vi "Main.vi"() -> ()   [LabVIEW 2021]
doc: "The myRIO Project template acquires acceleration data from the onboard accelerometer and displays the changes of acceleration values in a waveform chart."
uses:
  <vilib>/myRIO/Instrument Drivers/Onboard IO/I2C/typedefs/I2C User Configuration.ctl
  <vilib>/myRIO/Instrument Drivers/Onboard IO/I2C/typedefs/I2C Transfer Rate.ctl
  <vilib>/myRIO/Instrument Drivers/Onboard IO/I2C/typedefs/I2C Reference.ctl
  <vilib>/myRIO/Common/Instrument Driver Framework/Utilities/typedefs/myRIO Generic Hardware Reference.ctl
  <vilib>/myRIO/Common/Instrument Driver Framework/Utilities/typedefs/Hardware Version Enum.ctl
  <vilib>/myRIO/Common/Instrument Driver Framework/Utilities/typedefs/myRIO v1.0 Reference.ctl
  <vilib>/myRIO/Common/Instrument Driver Framework/Utilities/typedefs/Generic FPGA Reference.ctl
  <vilib>/myRIO/Common/Instrument Driver Framework/myRIO v1.0/I2C/typedefs/I2C Channels Enum.ctl
  <vilib>/myRIO/Instrument Drivers/Onboard IO/I2C/typedefs/I2C Configuration.ctl
  <vilib>/userDefined/High Color/nirio_resource_hc.ctl
  <vilib>/Platform/TimedLoop/XDataNode/timing_clust.ctl
  <vilib>/Platform/TimedLoop/XDataNode/nitl_modes.ctl
  <vilib>/Platform/TimedLoop/XDataNode/wakeup.ctl
  <vilib>/myRIO/Instrument Drivers/Onboard IO/PWM/typedefs/PWM Reference.ctl
  <vilib>/myRIO/Common/Instrument Driver Framework/myRIO v1.0/PWM/typedefs/PWM Channels Enum.ctl
  <vilib>/myRIO/Instrument Drivers/Onboard IO/PWM/typedefs/PWM Configuration.ctl
  <vilib>/myRIO/Common/Instrument Driver Framework/Utilities/vis/Is FPGA Ref Available.vi
  <vilib>/myRIO/Common/Instrument Driver Framework/myRIO v1.0/I2C/vis/myRIO v1.1 Open I2C.vi
  <vilib>/myRIO/Instrument Drivers/Onboard IO/I2C/vis/Configure.vi
  <vilib>/myRIO/Instrument Drivers/Onboard IO/I2C/vis/Write.vi
  <vilib>/myRIO/Instrument Drivers/Onboard IO/I2C/vis/Read.vi
  <vilib>/myRIO/Instrument Drivers/Onboard IO/I2C/vis/Write Read.vi
  <vilib>/myRIO/Common/Instrument Driver Framework/myRIO v1.0/PWM/vis/myRIO v1.1 Open PWM.vi
  <vilib>/myRIO/Instrument Drivers/Onboard IO/PWM/vis/Set Duty Cycle and Frequency.vi
  <vilib>/myRIO/Common/Instrument Driver Framework/Utilities/vis/Validate Channels.vi
  <vilib>/myRIO/Common/Instrument Driver Framework/myRIO v1.0/I2C/vis/myRIO v1.0 Reserve I2C.vi
  <vilib>/myRIO/Common/Instrument Driver Framework/myRIO v1.0/PWM/vis/myRIO v1.0 Reserve PWM.vi
  <vilib>/myRIO/Common/Instrument Driver Framework/myRIO v1.0/I2C/vis/myRIO v1.0 Build MUX Configuration I2C.vi
  <vilib>/myRIO/Common/Instrument Driver Framework/myRIO v1.0/Resource Manager/vis/myRIO v1.0 Reserve Channel List.vi
  <vilib>/myRIO/Common/Instrument Driver Framework/myRIO v1.0/PWM/vis/myRIO v1.0 Build MUX Configuration PWM.vi
  <vilib>/myRIO/Common/Instrument Driver Framework/myRIO v1.0/Resource Manager/vis/myRIO v1.0 Create Configuration List.vi
  <vilib>/myRIO/Common/Instrument Driver Framework/myRIO v1.0/Resource Manager/vis/myRIO v1.0 Reserve Channel.vi
  <vilib>/myRIO/Common/Instrument Driver Framework/myRIO v1.0/Resource Manager/vis/myRIO v1.0 Unreserve Channel.vi
  <vilib>/myRIO/Common/Instrument Driver Framework/myRIO v1.0/Resource Manager/vis/myRIO v1.0 Build Mutex Name.vi
  <vilib>/Utility/VariantDataType/GetNumericInfo.vi
  <vilib>/Utility/error.llb/Error Cluster From Error Code.vi
  <vilib>/myRIO/Common/Instrument Driver Framework/myRIO v1.0/myRIO v1.1 Open.vi
  <vilib>/myRIO/Common/Instrument Driver Framework/Utilities/vis/IO Manager.vi
  <vilib>/myRIO/Common/Instrument Driver Framework/Utilities/vis/Configuration Manager.vi
  <vilib>/myRIO/Common/Instrument Driver Framework/myRIO v1.0/Resource Manager/vis/myRIO v1.0 Configure IO.vi
  <vilib>/myRIO/Common/Instrument Driver Framework/myRIO v1.0/myRIO v1.0 Close.vi
  <vilib>/myRIO/Common/Instrument Driver Framework/myRIO v1.0/I2C/vis/myRIO v1.0 Configure I2C.vi
  <vilib>/myRIO/Common/Instrument Driver Framework/myRIO v1.0/I2C/vis/myRIO v1.0 Write I2C.vi
  <vilib>/myRIO/Common/Instrument Driver Framework/myRIO v1.0/I2C/vis/myRIO v1.0 Read I2C.vi
  <vilib>/myRIO/Common/Instrument Driver Framework/myRIO v1.0/PWM/vis/myRIO v1.0 Write PWM.vi
  <vilib>/Skyline/Tag/Wrapper/Wrapper_class/Close Tag (Multiple).vi
  <vilib>/Skyline/Tag/Wrapper/Wrapper_class/NI Skyline Tag.lvclass
  <vilib>/myRIO/Express VI/Onboard IO/I2C/I2C Express VI.xnode
  <vilib>/myRIO/Instrument Drivers/Onboard IO/I2C/vis/myRIO I2C Open.xnode
  <vilib>/platform/TimedLoop/XDataNode/XDataNode.xnode
  <vilib>/myRIO/Express VI/Onboard IO/PWM/PWM Express VI.xnode
  <vilib>/myRIO/Instrument Drivers/Onboard IO/PWM/vis/myRIO PWM Open.xnode
  <vilib>/myRIO/Instrument Drivers/Onboard IO/I2C/I2C.lvlib
  <vilib>/Platform/TimedLoop/XDataNode/XDNodeRunTimeDep.lvlib
  <vilib>/myRIO/Instrument Drivers/Onboard IO/PWM/PWM.lvlib
panel:
  out "Warmer\nON":bool
  out "Coffee Temp (°F)":dbl
  out "Error":errorcluster
  out "HOT\nSurface":bool
  out "Plate Temp (°F)":dbl
  out "Surface Danger Level":string
  out "Set-Temp-Slider":dbl(slide) scale=80.0..180.0
  out "Temp-Chart":T1(graph)
  in  "stop":bool
  # "Nice Warm Coffee"
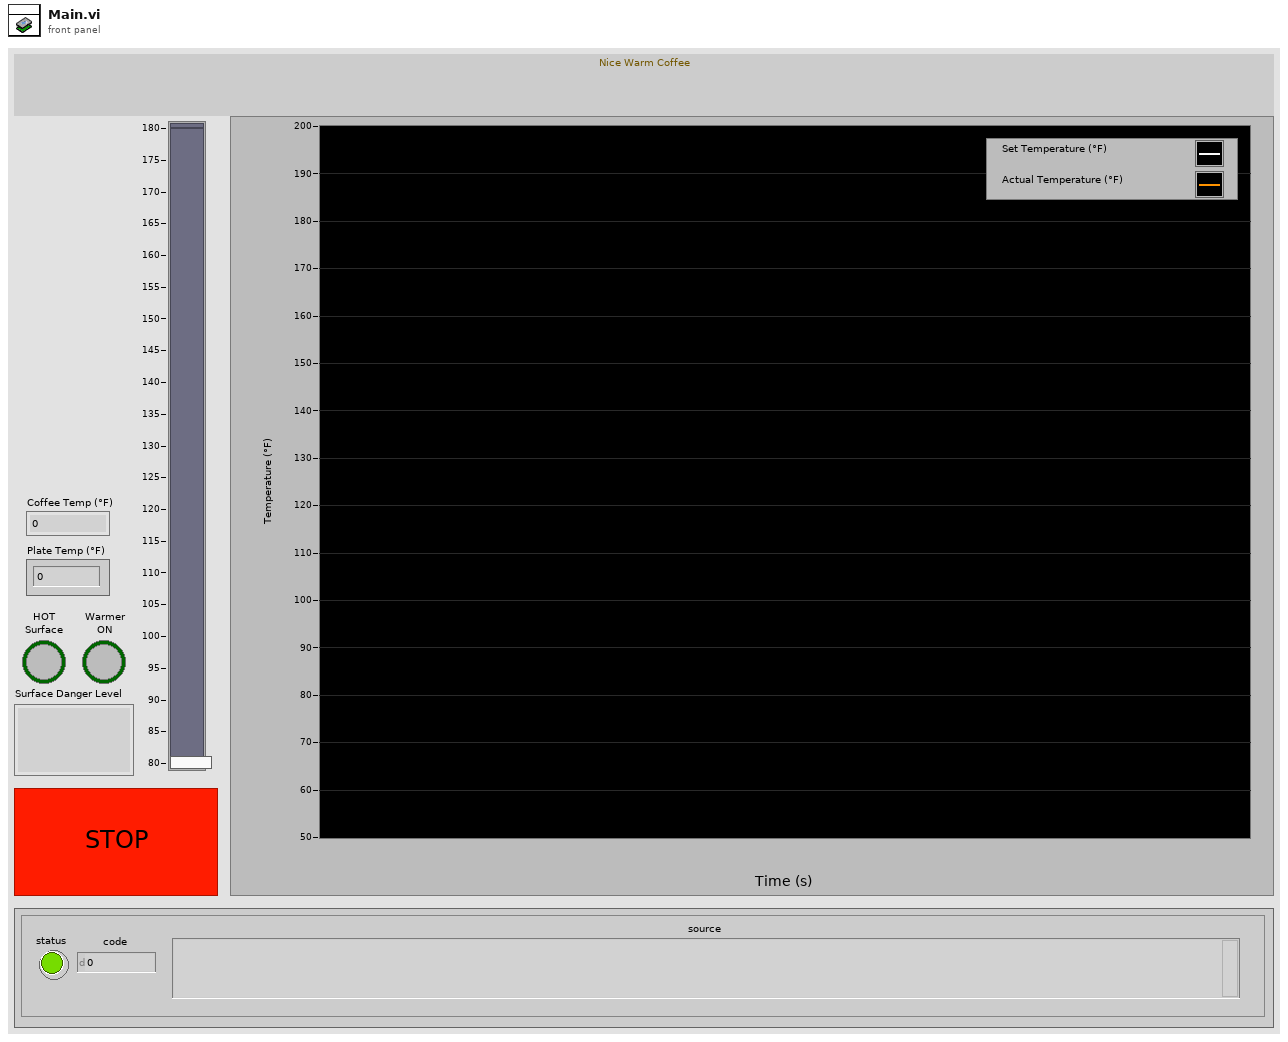
[diagram p1: front panel]
types:
  T1 = cluster{"[0]":dbl, "[1]":dbl, "[2]":dbl, "[3]":dbl, "[4]":dbl, "[5]":dbl, "[6]":dbl, "[7]":dbl, "[8]":dbl}
  T2 = typedef "XDNodeRunTimeDep.lvlib/timing_clust.ctl" = cluster{"Expected End [f-1]":u64, "Actual End [f-1]":u64, "Finished Late? [f-1]":bool, "Expected End [i-1]":u64, "Actual End [i-1]":u64, "Finished Late? [i-1]":bool, "Expected Start [i]":u64, "Actual Start [i]":u64, "Expected Start [f]":u64, "Actual Start [f]":u64, "Source Name":string, "Structure Name":string, "Period":i64, "Deadline":i64, "Offset":i64, "Start":i64, "Priority":i32, "Timeout":i32, "Mode":T3, "Wakeup Reason":T4, "Error":errorcluster, "Source Type":string, "Secondary Source Type":string, "Global End Time":u64, "Global Start Time":u64, "Frame Duration":u64, "Iteration Duration":u64, "Assigned CPU":i32, "I/O Scan Engine Mode":u32}
  T3 = typedef "XDNodeRunTimeDep.lvlib/nitl_modes.ctl" = enum32{"No Change", "Process missed periods, maintain original phase", "Discard missed periods, maintain original phase", "Process missed periods, ignore original phase", "Discard missed periods, ignore original phase"}
  T4 = typedef "XDNodeRunTimeDep.lvlib/wakeup.ctl" = enum32{"Normal", "Aborted", "Asynchronous wakeup", "Timing source error", "Timed loop error", "Timeout"}
  T5 = typedef "PWM.lvlib/PWM Reference.ctl" = cluster{"myRIO Reference":T6, "PWM Channels Enum":T10, "PWM Configuration":T11}
  T6 = typedef "myRIO Generic Hardware Reference.ctl" = cluster{"myRIO Model":T7, "myRIO Hardware Reference":T8}
  T7 = typedef "Hardware Version Enum.ctl" = enum16{"Unknown", "myRIO-1900", "myRIO-1950", "roboRIO", "NI ELVIS RIO CM", "ELVIS III"}
  T8 = typedef "myRIO v1.0 Reference.ctl" = cluster{"Generic FPGA Reference":T9, "Allow multiple opens":bool}
  T9 = typedef "Generic FPGA Reference.ctl" = refnum<k20>
  T10 = typedef "PWM Channels Enum.ctl" = enum16{"Not Connected", "C/PWM0", "C/PWM1", "A/PWM0", "A/PWM1", "A/PWM2", "A/PWM3", "A/PWM4", "A/PWM5", "A/PWM6", "A/PWM7", "A/PWM8", "A/PWM9", "A/PWM10", "A/PWM11", "A/PWM12", "A/PWM13", "A/PWM14", "A/PWM15", "A/PWM16", "A/PWM17", "A/PWM18", "A/PWM19", "B/PWM0", "B/PWM1", "B/PWM2", "B/PWM3", "B/PWM4", "B/PWM5", "B/PWM6", "B/PWM7", "B/PWM8", "B/PWM9", "B/PWM10", "B/PWM11", "B/PWM12", "B/PWM13", "B/PWM14", "B/PWM15", "B/PWM16", "B/PWM17", "B/PWM18", "B/PWM19", "PWM/PWM0", "PWM/PWM1", "PWM/PWM2", "PWM/PWM3", "PWM/PWM4", "PWM/PWM5", "PWM/PWM6", "PWM/PWM7", "PWM/PWM8", "PWM/PWM9"}
  T11 = typedef "PWM.lvlib/PWM Configuration.ctl" = cluster{"Frequency":dbl, "Duty Cycle":dbl}
  T12 = typedef "nirio_resource_hc.ctl" = tag
  T13 = typedef "I2C.lvlib/I2C Reference.ctl" = cluster{"myRIO Reference":T6, "I2C Channels Enum":T14, "I2C Configuration":T15}
  T14 = typedef "I2C Channels Enum.ctl" = enum16{"Not Connected", "A/I2C", "B/I2C", "I2C/I2C"}
  T15 = typedef "I2C.lvlib/I2C Configuration.ctl" = cluster{"I2C Transfer Rate":T16}
  T16 = typedef "I2C.lvlib/I2C Transfer Rate.ctl" = enum16{"Standard mode (100 kbps)", "Fast mode (400 kbps)"}
  T17 = typedef "I2C.lvlib/I2C User Configuration.ctl" = cluster{"I2C Transfer Rate":T16}
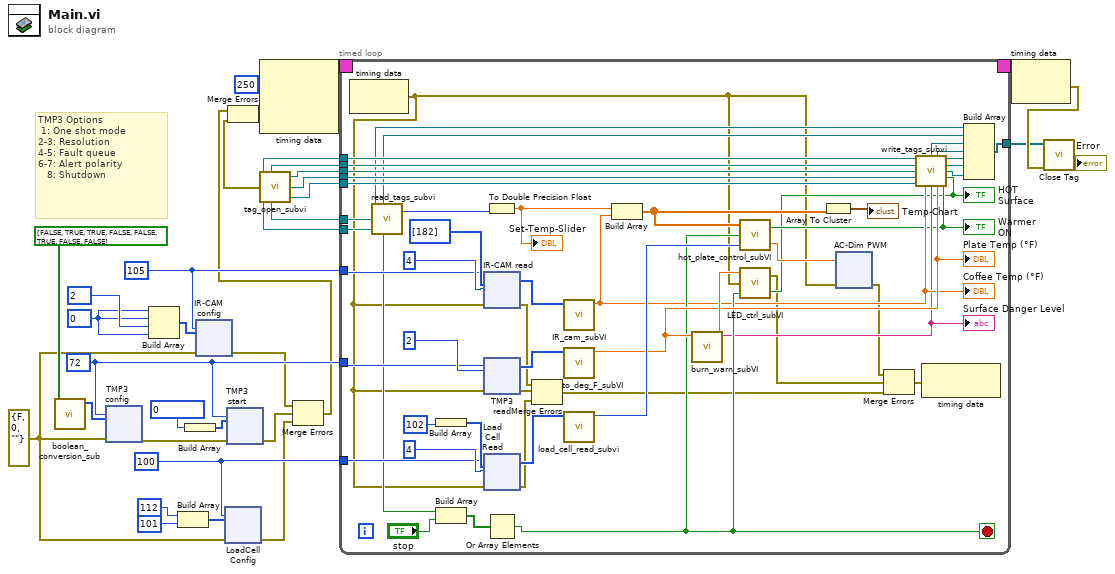
[diagram p0: block diagram]
diagram:
  w18 = errorcluster {"status"=FALSE, "code"=0, "source"=""} ("error in (no error)")
  w23 = u8 100 ("Slave Address (7-bit)")
  w1 = u8 0
  w21 = u8 105 ("Slave Address (7-bit)")
  w22 = u8 72 ("Slave Address (7-bit)")
  # "TMP3 Options  \n 1: One shot mode\n2-3: Resolution \n4-5: Fault queue\n6-7: Alert polarity\n   8: Shutdown"
  n1 = call "boolean_conversion_sub.vi"("Array in"=bool[] [FALSE, TRUE, TRUE, FALSE, FALSE, TRUE, FALSE, FALSE]) -> ("Array out"=w33:u8[])  [unwired: 10 in]
  n2 = xnode "TMP3\nconfig"("error in (no error)"=w18, "Slave Address (7-bit)"=w22, "Bytes to Write"=w33) -> ("error out"=w19:errorcluster)
  n3 = Build Array(w1, w1, u8 2, w1) -> (w30:u8[])
  n4 = Build Array(u8 112 ("Slave Address (7-bit)"), u8 101 ("Slave Address (7-bit)")) -> (w27:u8[])
  n5 = Build Array(u8 0) -> (w31:u8[])
  n6 = xnode "IR-CAM\nconfig"("error in (no error)"=w18, "Slave Address (7-bit)"=w21, "Bytes to Write"=w30) -> ("error out"=w4:errorcluster)
  n7 = xnode "LoadCell\nConfig"("error in (no error)"=w18, "Slave Address (7-bit)"=w23, "Bytes to Write"=w27) -> ("error out"=w3:errorcluster)
  n8 = xnode "TMP3\nstart"("error in (no error)"=w19, "Slave Address (7-bit)"=w22, "Bytes to Write"=w31) -> ("error out"=w5:errorcluster)
  n9 = call "tag_open_subvi.vi"() -> ("Warn String"=w14:refnum<class "NI Skyline Tag.lvclass">, "Plate-ON"=w13:refnum<class "NI Skyline Tag.lvclass">, "error out"=w6:errorcluster, "STOPWEB"=w7:refnum<class "NI Skyline Tag.lvclass">, "User-T"=w8:refnum<class "NI Skyline Tag.lvclass">, "Hot-Sfc"=w12:refnum<class "NI Skyline Tag.lvclass">, "Plate-T"=w11:refnum<class "NI Skyline Tag.lvclass">, "Coffee-T"=w10:refnum<class "NI Skyline Tag.lvclass">)
  n10 = Merge Errors(w4, w5, w3) -> (w2:errorcluster)
  n11 = Merge Errors(w2, w6) -> (w17:errorcluster)
  n12 = node-c288(i64 250 ("Period"), w17) -> (w25:T2)  [unwired: 1 in]
  n13 = timed-loop {
    timing: w25 -> [_]
    timing-out: [_] -> w24
    tunnel: w23 -> [w74]
    tunnel: w22 -> [w73]
    tunnel: w21 -> [w72]
    tunnel: w14 -> [w65]
    tunnel: w13 -> [w64]
    tunnel: w12 -> [w63]
    tunnel: w11 -> [w62]
    tunnel: w10 -> [w61]
    tunnel: [w60] -> w9
    tunnel: w8 -> [w42]
    tunnel: w7 -> [w41]
    stop <- w67 stop-if-true
    n14 = node-c288() -> (w35:errorcluster)  [unwired: 1 in]
    n15 = call "read_tags_subvi.vi"("USER-T-in"=w42, "STOP-in"=w41) -> ("USER-T-out"=w50:refnum<class "NI Skyline Tag.lvclass">, "STOP-out"=w51:refnum<class "NI Skyline Tag.lvclass">, "StopWeb"=w40:bool, "User-T-int"=w55:i32)  [unwired: 1 in]
    n16 = Build Array(u8 102 ("Slave Address (7-bit)")) -> (w83:u8[])
    n17 = Build Array(w40, "stop") -> (w66:bool[])
    n18 = xnode "IR-CAM read"("error in (no error)"=w35, "Slave Address (7-bit)"=w72, "Bytes to Write"=u8[] [182], "Byte Count"=u32 4) -> ("error out"=w59:errorcluster, "Bytes Read"=w79:u8[])
    n19 = xnode "TMP3\nread"("error in (no error)"=w35, "Slave Address (7-bit)"=w73, "Byte Count"=u32 2) -> ("error out"=w58:errorcluster, "Bytes Read"=w77:u8[])
    n20 = xnode "Load\nCell\nRead"("error in (no error)"=w35, "Slave Address (7-bit)"=w74, "Bytes to Write"=w83, "Byte Count"=u32 4) -> ("error out"=w57:errorcluster, "Bytes Read"=w85:u8[])
    n21 = To Double Precision Float(number=w55) -> (double precision float=w53:dbl)
    "Set-Temp-Slider" <- w53
    n22 = Or Array Elements(Boolean array=w66) -> (logical OR=w67:bool)
    n23 = Merge Errors(w59, w58, w57) -> (w37:errorcluster)
    n24 = call "IR_cam_subVI.vi"("Bytes Read"=w79) -> ("Numeric"=w54:dbl)  [unwired: 10 in]
    "Coffee Temp (°F)" <- w54
    n25 = call "to_deg_F_subVI.vi"("Bytes Read"=w77) -> ("Numeric"=w68:dbl)  [unwired: 10 in]
    "Plate Temp (°F)" <- w68
    n26 = call "load_cell_read_subvi.vi"("Bytes Read"=w85) -> ("Numeric"=w69:u32)  [unwired: 10 in]
    n27 = Build Array(w53, w54) -> (w71:dbl[])
    n28 = call "burn_warn_subVI.vi"("Placeholder\nSfc Temp"=w68) -> ("Level"=w76:dbl, "String"=w52:string)  [unwired: 9 in]
    "Surface Danger Level" <- w52
    n29 = call "hot_plate_control_subVI.vi"("LoadCell"=w69, "Stop-button"=w67, "Array"=w71) -> ("Numeric"=w70:dbl, "Warmer\nON"=w44:bool)
    "Warmer\nON" <- w44
    n30 = call "LED_ctrl_subVI.vi"("stop"=w67, "error in (no error)"=w35, "Numeric in"=w76) -> ("HOT\nSurface"=w43:bool, "error out"=w38:errorcluster)
    "HOT\nSurface" <- w43
    n31 = Array To Cluster(array=w71) -> (cluster=→"Temp-Chart":T1)
    n32 = xnode "AC-Dim PWM"("error in (no error)"=w35, "Duty Cycle"=w70) -> ("error out"=w39:errorcluster)
    n33 = Merge Errors(w39, w38, w37) -> (w36:errorcluster)
    n34 = call "write_tags_subvi.vi"(0:"Warn String"=w65, "Plate ON"=w64, "Hot-Sfc"=w63, 9:"Plate-T"=w62, "HOT\nSurface"=w43, 11:"Coffee-T"=w61, 12:"Coffee-T"=w54, 13:"Warn String"=w52, 14:"Plate-T"=w68, "Warmer\nON"=w44) -> ("tag out"=w49:refnum<class "NI Skyline Tag.lvclass">, "tag out 2"=w48:refnum<class "NI Skyline Tag.lvclass">, "NI Skyline Tag out"=w47:refnum<class "NI Skyline Tag.lvclass">, "tag out 4"=w46:refnum<class "NI Skyline Tag.lvclass">, "tag out 3"=w45:refnum<class "NI Skyline Tag.lvclass">)  [unwired: 1 in]
    n35 = node-c288(w36) -> ()  [unwired: 1 out]
    n36 = Build Array(w50, w51, w49, w48, w47, w46, w45) -> (w60:refnum<class "NI Skyline Tag.lvclass">[])
  }
  n37 = node-c288(w24) -> (w16:errorcluster)
  n38 = call-poly <vilib>:"Close Tag.vi"("error in (no error)"=w16, "tags"=w9) -> ("error out"=→"Error":errorcluster)  [unwired: 9 in]
